vi "Set Plot Names.vi"(8 "error in":errorcluster, 10 "Plot Names":string[](array[string]), 11 "Graph Reference":refnum<vi>) -> (0 "error out":errorcluster)   [LabVIEW 2012]
doc: "This VI is used to set the plot names on a Waveform Chart or Waveform Graph."
uses:
  <vilib>/Utility/error.llb/Error Cluster From Error Code.vi
  <vilib>/ErrorRing/Error Ring.xnode
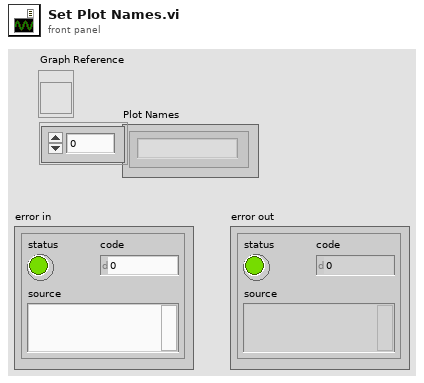
[diagram p1: front panel]
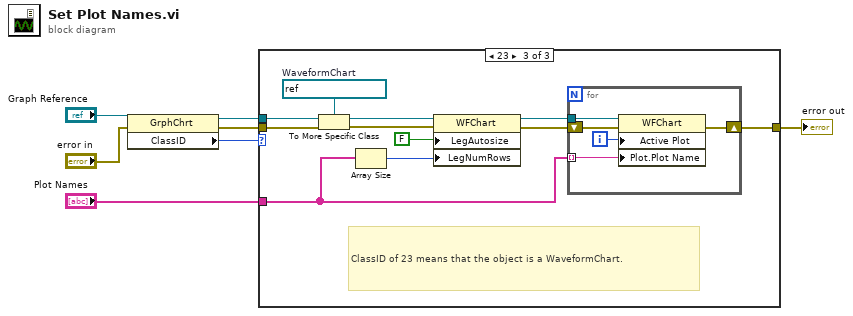
[diagram p0: block diagram]
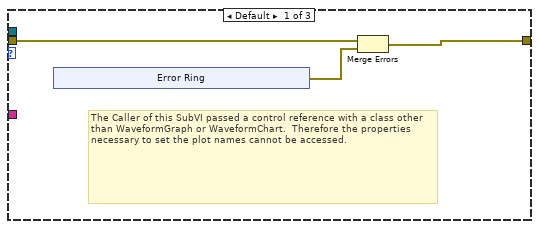
[diagram p2: hidden frame]
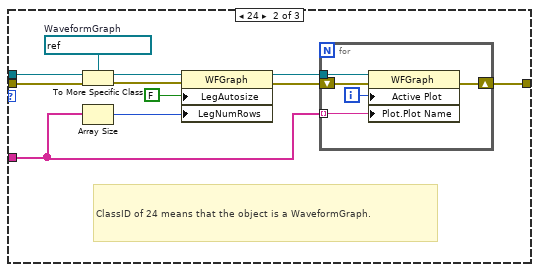
[diagram p3: hidden frame]
diagram:
  n1 = property class="GrphChrt"(reference="Graph Reference", error in="error in") -> (reference out=w5:refnum<vi>, error out=w6:errorcluster, "ClassID"=w1:u32)
  n2 = case shown="23" w1 {
    tunnel: w6 -> [w10 w19 w35]
    tunnel: w5 -> [_ w20 w36]
    tunnel: "Plot Names" -> [_ w15 w31]
    tunnel: [w9 w17 w33] -> w3
    frame Default {
      # "The Caller of this SubVI passed a control reference with a class other than WaveformGraph or WaveformChart.  Therefore the properties necessary to set the plot names cannot be accessed."
      n3 = xnode "Error Ring"() -> ("error out"=w8:errorcluster)
      n4 = Merge Errors(w10, w8) -> (w9:errorcluster)
    }
    frame 24 {
      w25 = refnum<vi> refnum  # WaveformGraph
      # "ClassID of 24 means that the object is a WaveformGraph."
      n5 = To More Specific Class(target class=w25, reference=w20, error in=w19) -> (specific class reference=w23:refnum<vi>, error out=w24:errorcluster)
      n6 = Array Size(array=w15) -> (size(s)=w16:i32)
      n7 = property class="WFGraph"(reference=w23, error in=w24, "LegAutosize"=FALSE ("Legend:Autosize"), "LegNumRows"=w16) -> (reference out=w21:refnum<vi>, error out=w18:errorcluster)
      n8 = for {
        tunnel: w21 -> [w30]
        shift-right: [w28] -> w17
        shift-left: w18 -> [w29]
        tunnel: w15 -> [w26] mode=indexing
        i -> [w27]
        n9 = property class="WFGraph"(reference=w30, error in=w29, "Active Plot"=w27, "Plot.Plot Name"=w26) -> (error out=w28:errorcluster)  [unwired: 1 out]
      }
    }
    frame 23 {
      w41 = refnum<vi> refnum  # WaveformChart
      # "ClassID of 23 means that the object is a WaveformChart."
      n10 = To More Specific Class(target class=w41, reference=w36, error in=w35) -> (specific class reference=w39:refnum<vi>, error out=w40:errorcluster)
      n11 = Array Size(array=w31) -> (size(s)=w32:i32)
      n12 = property class="WFChart"(reference=w39, error in=w40, "LegAutosize"=FALSE ("Legend:Autosize"), "LegNumRows"=w32) -> (reference out=w37:refnum<vi>, error out=w34:errorcluster)
      n13 = for {
        tunnel: w37 -> [w46]
        shift-right: [w44] -> w33
        shift-left: w34 -> [w45]
        tunnel: w31 -> [w42] mode=indexing
        i -> [w43]
        n14 = property class="WFChart"(reference=w46, error in=w45, "Active Plot"=w43, "Plot.Plot Name"=w42) -> (error out=w44:errorcluster)  [unwired: 1 out]
      }
    }
  }
  "error out" <- w3
